vi "Begin.vi"(8 "error in":errorcluster) -> (0 "error out":errorcluster)   [LabVIEW 2014]
doc: "Called before other user functions, this VI is expected to open initial I/O refnums, load in file data, and do all program initialization. Notice that the <B>error out</B> terminal is simply used for data flow. Wiring it to other structures or subVIs ensures that this VI runs first."
uses:
  <vilib>/Rock Robotics/WPI/SafetyOutput/WPI_SafetyOutputConfigMenu.ctl
  <vilib>/Rock Robotics/WPI/DriverStation/WPI_DriverStationRobotMode2.ctl
  <vilib>/Rock Robotics/WPI/Joystick/WPI_JoystickDeviceEnum.ctl
  <vilib>/Rock Robotics/WPI/Solenoid/WPI_SolenoidChannel.ctl
  <vilib>/Rock Robotics/SystemInterfaces/DIO/FPGA_DIOChannel.ctl
  Robot Global Data.vi
  <vilib>/Rock Robotics/Network Tables/SD Write String Array.vi
  <vilib>/Rock Robotics/WPI/RobotDrive/WPI_RobotDriveOpen2MotorWithCANTalonSRX.vi
  <vilib>/Rock Robotics/WPI/MotorControl/WPI_MotorControlOpenCANTalonSRX.vi
  <vilib>/Rock Robotics/WPI/Solenoid/WPI_SolenoidOpenDouble.vi
  <vilib>/Rock Robotics/WPI/Compressor/WPI_CompressorGetSetRefNum.vi
  <vilib>/Rock Robotics/WPI/Switch/WPI_SwitchOpenLimit.vi
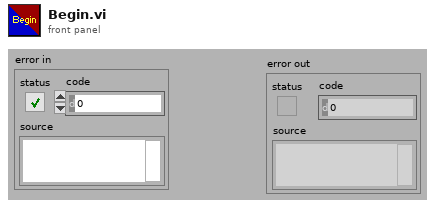
[diagram p1: front panel]
types:
  T1 = typedef "FPGA_DIOChannel.ctl" = enum8{"DIO 0", "DIO 1", "DIO 2", "DIO 3", "DIO 4", "DIO 5", "DIO 6", "DIO 7", "DIO 8", "DIO 9", "DIO MXP 0", "DIO MXP 1", "DIO MXP 2", "DIO MXP 3", "DIO MXP 4", "DIO MXP 5", "DIO MXP 6", "DIO MXP 7", "DIO MXP 8", "DIO MXP 9", "DIO MXP 10", "DIO MXP 11", "DIO MXP 12", "DIO MXP 13", "DIO MXP 14", "DIO MXP 15", "Invalid"}
  T2 = typedef "WPI_SolenoidChannel.ctl" = enum8{"Solenoid 0", "Solenoid 1", "Solenoid 2", "Solenoid 3", "Solenoid 4", "Solenoid 5", "Solenoid 6", "Solenoid 7", "Invalid"}
  T3 = typedef "WPI_JoystickDeviceEnum.ctl" = enum16{"USB 0", "USB 1", "USB 2", "USB 3", "USB 4", "USB 5"}
  T4 = typedef "WPI_DriverStationRobotMode2.ctl" = enum16{"Autonomous Disabled", "Autonomous Enabled", "Teleop Disabled", "Teleop Enabled", "Disconnected", "Finish", "Test Disabled", "Test Enabled", "Emergency Stopped"}
  T5 = typedef "WPI_SafetyOutputConfigMenu.ctl" = enum16{"Enable", "Disable"}
  T6 = typedef "WPI_SolenoidDevRef.ctl" = cluster{"DevStatus":errorcluster, "Pneumatics Control Module":u8, "Forward Solenoid Channel":T2, "Reverse Solenoid Channel":T2}
  T7 = typedef "WPI_SwitchDevRef.ctl" = cluster{"DevStatus":errorcluster, "DIO Channel":T1, "Controller":T8, "CntIndex":T9, "Normally Closed":bool}
  T8 = typedef "FPGA_TypedefDigitalModule.ctl" = enum16{"Controller 1"}
  T9 = typedef "FPGA_CounterCtrSystemIndex.ctl" = enum8{"Ctr 0", "Ctr 1", "Ctr 2", "Ctr 3", "Ctr 4", "Ctr 5", "Ctr 6", "Ctr 7", "Invalid"}
  T10 = typedef "WPI_CompressorDevRef.ctl" = cluster{"DevStatus":errorcluster, "Pneumatics Control Module":u8}
  T11 = typedef "WPI_MotorControlDeviceRef.ctl" = cluster{"DeviceStatus":errorcluster, "Type":T12, "PWM":cluster{"Controller":T8, "PWM Channel":T13, "DeadBand":T14}, "CAN":cluster{"Device Number":u8, "Control Mode":T15, "Semaphore":T16, "Max Vout":dbl, "TalonSRX Control Mode":T17}, "Invert":bool, "TransformRef":T18, "InvTransformRef":T18}
  T12 = typedef "WPI_MotorControlType.ctl" = enum16{"PWM", "CAN", "CANTalonSRX"}
  T13 = typedef "FPGA_DIOPWMChannel.ctl" = enum8{"PWM 0", "PWM 1", "PWM 2", "PWM 3", "PWM 4", "PWM 5", "PWM 6", "PWM 7", "PWM 8", "PWM 9", "PWM MXP 0", "PWM MXP 1", "PWM MXP 2", "PWM MXP 3", "PWM MXP 4", "PWM MXP 5", "PWM MXP 6", "PWM MXP 7", "PWM MXP 8", "PWM MXP 9", "Invalid"}
  T14 = typedef "WPI_PWMDeadband.ctl" = cluster{"Name":string, "maxPositivePwm":i32, "minPositivePwm":i32, "centerPwm":i32, "maxNegativePwm":i32, "minNegativePwm":i32, "angularRange":u16}
  T15 = typedef "WPI_CANJaguar_ControlMode.ctl" = enum8{"Percent VBus", "Current", "Speed", "Position", "Voltage"}
  T16 = typedef "Semaphore RefNum" = refnum<k1>
  T17 = typedef "WPI_CANTalonSRX_APIControlMode.ctl" = enum8{"Percent VBus", "Speed", "Position", "Slave", "Unchanged / Invalid"}
  T18 = typedef "WPI_PWMTransform_ConPane.ctl" = refnum<vi>
  T19 = typedef "WPI_JoystickDevRef.ctl" = cluster{"Device":T3}
  T20 = typedef "WPI_RobotDriveDevRef.ctl" = cluster{"DevStatus":errorcluster, "Motors[]":T11[], "Square Inputs":bool, "Max Output":dbl}
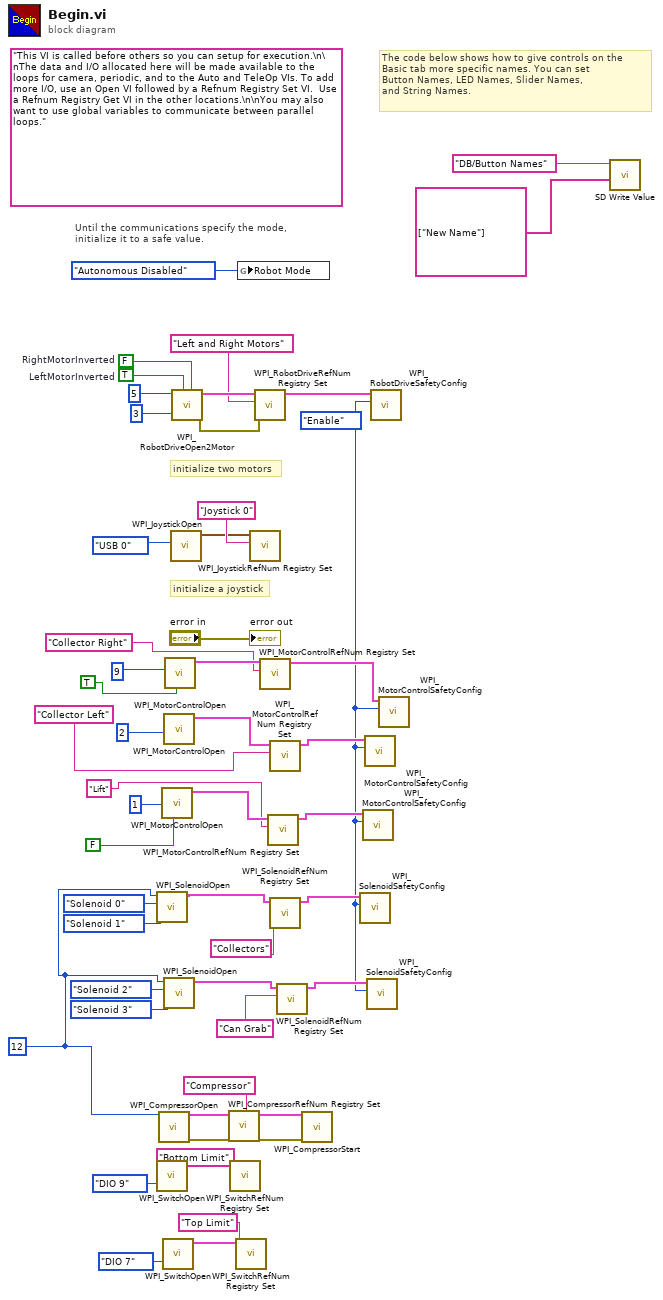
[diagram p0: block diagram]
diagram:
  w9 = u8 12 ("Pneumatics Control Module (0)")
  w19 = WPI_SafetyOutputConfigMenu."Enable" ("mode")
  (unwired) "This VI is called before others so you can setup for execution.\n\nThe data and I/O allocated here will be made available to the loops for camera, periodic, and to the Auto and TeleOp VIs. To add more I/O, use an Open VI followed by a Refnum Registry Set VI.  Use a Refnum Registry Get VI in the other locations.\n\nYou may also want to use global variables to communicate between parallel loops."
  w51 = TRUE  # LeftMotorInverted
  w52 = FALSE  # RightMotorInverted
  # "The code below shows how to give controls on the\nBasic tab more specific names. You can set\nButton Names, LED Names, Slider Names,\nand String Names."
  # "initialize a joystick"
  # "Until the communications specify the mode,\ninitialize it to a safe value."
  # "initialize two motors"
  n1 = call-poly <vilib>:"WPI_SolenoidOpen.vi"("Reverse Solenoid Channel"=WPI_SolenoidChannel."Solenoid 1", "Forward Solenoid Channel"=WPI_SolenoidChannel."Solenoid 0", "Pneumatics Control Module (0)"=w9) -> ("SolenoidDevRef"=w23:T6)  [unwired: 7 in, 1 out]
  n2 = call-poly <vilib>:"WPI_SwitchOpen.vi"("DIO Channel"=FPGA_DIOChannel."DIO 9") -> ("SwitchDevRef"=w7:T7)  [unwired: 9 in, 1 out]
  n3 = call <vilib>:"WPI_CompressorOpen.vi"("Pneumatics Control Module (0)"=w9) -> ("CompressorDevRef"=w13:T10, "error out"=w14:errorcluster)  [unwired: 13 in]
  n4 = call-poly <vilib>:"WPI_MotorControlOpen.vi"("Invert"=FALSE, "Device Number"=u8 1) -> ("MotorControlDeviceRef"=w33:T11)  [unwired: 8 in, 1 out]
  n5 = call-poly <vilib>:"WPI_SwitchOpen.vi"("DIO Channel"=FPGA_DIOChannel."DIO 7") -> ("SwitchDevRef"=w4:T7)  [unwired: 9 in, 1 out]
  n6 = call-poly <vilib>:"WPI_MotorControlOpen.vi"("Device Number"=u8 2) -> ("MotorControlDeviceRef"=w38:T11)  [unwired: 9 in, 1 out]
  n7 = call-poly <vilib>:"WPI_SolenoidOpen.vi"("Reverse Solenoid Channel"=WPI_SolenoidChannel."Solenoid 3", "Forward Solenoid Channel"=WPI_SolenoidChannel."Solenoid 2", "Pneumatics Control Module (0)"=w9) -> ("SolenoidDevRef"=w21:T6)  [unwired: 7 in, 1 out]
  n8 = call-poly <vilib>:"WPI_MotorControlOpen.vi"("Invert"=TRUE, "Device Number"=u8 9) -> ("MotorControlDeviceRef"=w39:T11)  [unwired: 8 in, 1 out]
  n9 = call <vilib>:"WPI_JoystickOpen.vi"("JoystickDevice"=WPI_JoystickDeviceEnum."USB 0") -> ("JoystickDevRef"=w44:T19)  [unwired: 10 in]
  n10 = call-poly <vilib>:"WPI_RobotDriveOpen2Motor.vi"("Right Motor Inverted"=w52, "Left Motor Inverted"=w51, "Right Motor"=u8 3, "Left Motor"=u8 5) -> ("error out"=w48:errorcluster, "RobotDriveDevRef"=w50:T20)  [unwired: 1 in, 5 out]
  n11 = call <vilib>:"WPI_SwitchRefNum Registry Set.vi"("refnum name"="Bottom Limit", "SwitchDevRef"=w7) -> ()  [unwired: 8 in, 2 out]
  n12 = call <vilib>:"WPI_SwitchRefNum Registry Set.vi"("refnum name"="Top Limit", "SwitchDevRef"=w4) -> ()  [unwired: 8 in, 2 out]
  n13 = global write "Robot Global Data.vi" "Robot Mode"(WPI_DriverStationRobotMode2."Autonomous Disabled" ("Robot Mode")) -> ()
  n14 = call <vilib>:"WPI_JoystickRefNum Registry Set.vi"("refnum name"="Joystick 0", "JoystickDevRef"=w44) -> ()  [unwired: 8 in, 2 out]
  n15 = call <vilib>:"WPI_RobotDriveRefNum Registry Set.vi"("error in (no error)"=w48, "refnum name"="Left and Right Motors", "RobotDriveDevRef"=w50) -> ("RobotDriveDevRef"=w47:T20)  [unwired: 8 out]
  n16 = call <vilib>:"WPI_MotorControlRefNum Registry Set.vi"("refnum name"="Collector Right", "MotorControlDevRef"=w39) -> ("MotorControlDevRef"=w36:T11)  [unwired: 8 in, 1 out]
  n17 = call <vilib>:"WPI_MotorControlRefNum Registry Set.vi"("refnum name"="Lift", "MotorControlDevRef"=w33) -> ("MotorControlDevRef"=w32:T11)  [unwired: 8 in, 1 out]
  n18 = call <vilib>:"WPI_MotorControlRefNum Registry Set.vi"("refnum name"="Collector Left", "MotorControlDevRef"=w38) -> ("MotorControlDevRef"=w37:T11)  [unwired: 8 in, 1 out]
  n19 = call <vilib>:"WPI_SolenoidRefNum Registry Set.vi"("refnum name"="Collectors", "SolenoidDevRef"=w23) -> ("SolenoidDevRef"=w22:T6)  [unwired: 8 in, 1 out]
  n20 = call <vilib>:"WPI_SolenoidRefNum Registry Set.vi"("refnum name"="Can Grab", "SolenoidDevRef"=w21) -> ("SolenoidDevRef"=w20:T6)  [unwired: 8 in, 1 out]
  n21 = call <vilib>:"WPI_CompressorStart.vi"("error in (no error)"=w14, "CompressorDevRef"=w13) -> ("error out"=w12:errorcluster, "CompressorDevRef"=w11:T10)  [unwired: 8 in]
  n22 = call <vilib>:"WPI_CompressorRefNum Registry Set.vi"("error in (no error)"=w12, "refnum name"="Compressor", "CompressorDevRef"=w11) -> ()  [unwired: 7 in, 2 out]
  n23 = call <vilib>:"WPI_SolenoidSafetyConfig.vi"("mode"=w19, "SolenoidDevRef"=w22) -> ()  [unwired: 8 in, 2 out]
  n24 = call <vilib>:"WPI_MotorControlSafetyConfig.vi"("mode"=w19, "MotorControlDevRef"=w32) -> ()  [unwired: 8 in, 2 out]
  n25 = call <vilib>:"WPI_MotorControlSafetyConfig.vi"("mode"=w19, "MotorControlDevRef"=w37) -> ()  [unwired: 8 in, 2 out]
  n26 = call <vilib>:"WPI_SolenoidSafetyConfig.vi"("mode"=w19, "SolenoidDevRef"=w20) -> ()  [unwired: 8 in, 2 out]
  n27 = call <vilib>:"WPI_RobotDriveSafetyConfig.vi"("mode"=w19, "RobotDriveDevRef"=w47) -> ()  [unwired: 8 in, 2 out]
  n28 = call <vilib>:"WPI_MotorControlSafetyConfig.vi"("mode"=w19, "MotorControlDevRef"=w36) -> ()  [unwired: 8 in, 2 out]
  n29 = call-poly <vilib>:"SD Write Value.vi"("String Array"=string[] ["New Name"], "Name"="DB/Button Names") -> ()  [unwired: 8 in, 2 out]
  "error out" <- "error in"
